vi "configureAcquisition.vi"(6 "imagePaths":path[](array[path]), 7 "saveImages?":bool, 8 "error in (no error)":errorcluster, 9 "number of Images":i32, 10 "CameraSettings":refnum<class "CamaraSettings.lvclass">, 11 "Pixelfly in":refnum<class "Pixelfly.lvclass">) -> (0 "error out":errorcluster, 3 "Pixelfly out":refnum<class "Pixelfly.lvclass">)   [LabVIEW 2009, in "Hardware.lvlib" / "Channels.lvlib" / "Pixelfly.lvclass"]
uses:
  Pixelfly.lvclass
  Tools/CameraSettings/CamaraSettings.lvclass
  Tools/CameraSettings/PixelFlySettings/PixelflySettings.lvclass
  Pixelfly.lvclass/Pixelfly.ctl
  Camera.lvclass
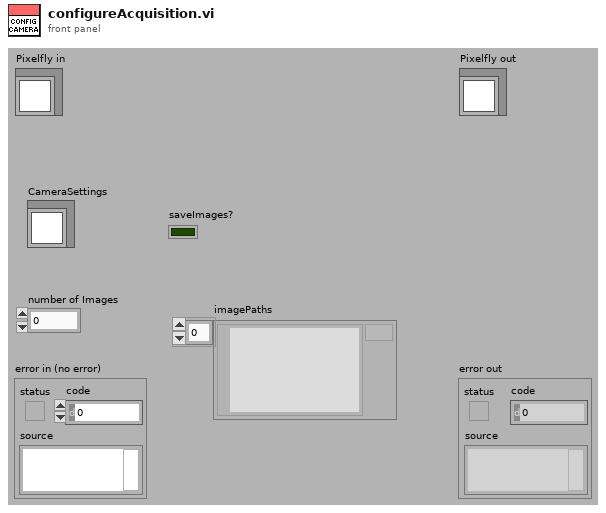
[diagram p1: front panel]
types:
  T1 = cluster{"ccdxsize":i32, "ccdy":i32, "pictx":i32, "picty":i32, "bitspixel":i32}
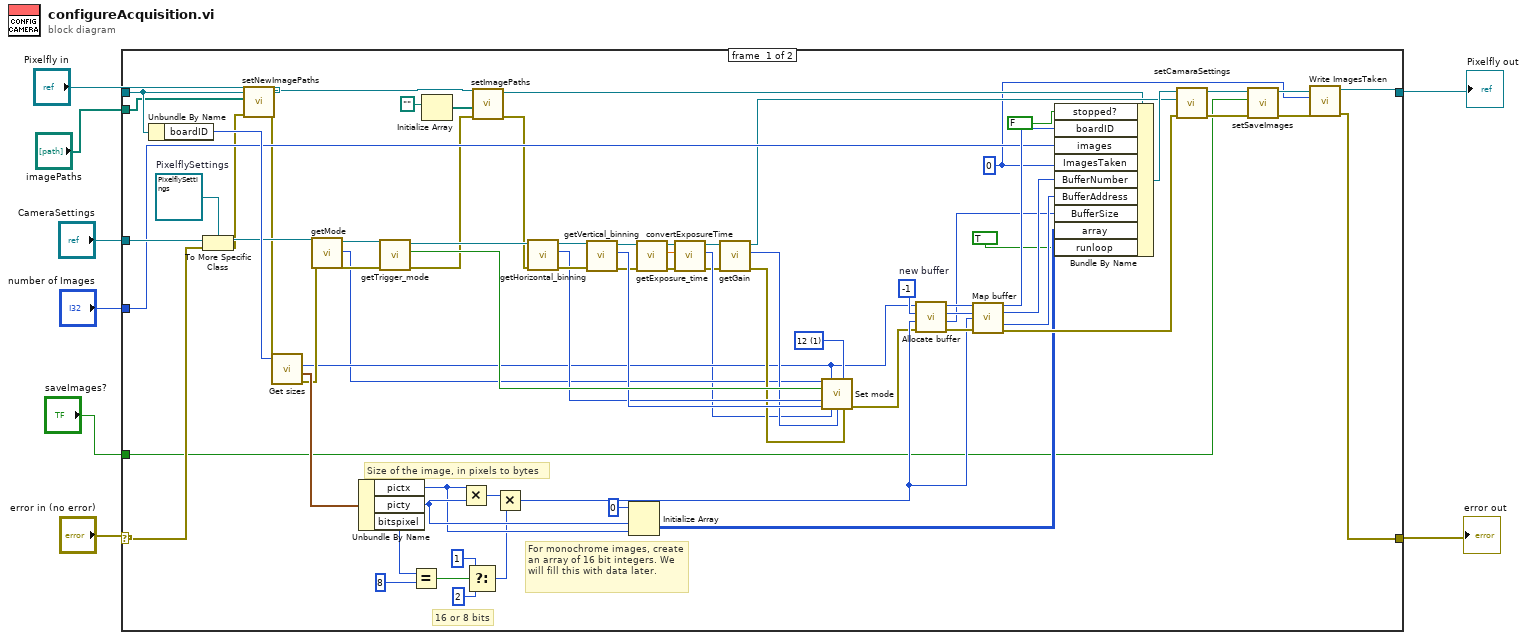
[diagram p0: block diagram]
diagram:
  n1 = case shown="No Error" "error in (no error)" {
    selector: "error in (no error)" -> [w79 w82]
    tunnel: "Pixelfly in" -> [w34 w83]
    tunnel: [w13 w83] -> w4
    tunnel: [w11 w82] -> w3
    tunnel: "CameraSettings" -> [w81 _]
    tunnel: "number of Images" -> [w42 _]
    tunnel: "imagePaths" -> [w31 _]
    tunnel: "saveImages?" -> [w22 _]
    frame #0 {
      w10 = 0
      w60 = 1 items=["8", "12"] ("bits/pixel")
      w63 = -1  # new buffer
      w80 = refnum<class "PixelflySettings.lvclass"> refnum  # PixelflySettings
      # "16 or 8 bits"
      # "For monochrome images, create an array of 16 bit integers. We will fill this with data later."
      # "Size of the image, in pixels to bytes"
      n2 = Unbundle By Name(w34) -> ("boardID"=w61:i32)
      n3 = To More Specific Class(target class=w80, reference=w81, error in=w79) -> (specific class reference=w59:refnum<class "PixelflySettings.lvclass">, error out=w33:errorcluster)
      n4 = call "setNewImagePaths.vi"("error in (no error)"=w33, "NewImagePaths"=w31, "Camera in"=w34) -> ("error out"=w32:errorcluster, "Camera out"=w30:refnum<class "Pixelfly.lvclass">)  [unwired: 7 in]
      n5 = call <instrlib>:"Get sizes.vi"("Handle in"=w61, "error in (no error)"=w32) -> ("Handle out"=w45:i32, "Picture parameters"=w73:T1, "error out"=w58:errorcluster)  [unwired: 1 in, 1 out]
      n6 = call "getMode.vi"("error in (no error)"=w58, "PixelflySettings in"=w59) -> ("error out"=w56:errorcluster, "mode"=w43:u16, "PixelflySettings out"=w57:refnum<class "PixelflySettings.lvclass">)  [unwired: 7 in]
      n7 = Unbundle By Name(w73) -> ("pictx"=w70:i32, "picty"=w71:i32, "bitspixel"=w72:i32)
      n8 = call "getTrigger_mode.vi"("error in (no error)"=w56, "PixelflySettings in"=w57) -> ("error out"=w27:errorcluster, "trigger_mode"=w55:bool, "PixelflySettings out"=w54:refnum<class "PixelflySettings.lvclass">)  [unwired: 7 in]
      n9 = Equal?(x=w72, y=8) -> (x = y?=w69:bool)
      n10 = Initialize Array(path "") -> (w28:path[])  [unwired: 1 in]
      n11 = Multiply(x=w70, y=w71) -> (x*y=w75:i32)
      n12 = Select(t=1, s=w69, f=2) -> (s? t:f=w66:i32)
      n13 = call "setImagePaths.vi"("error in (no error)"=w27, "ImagePaths"=w28, "Camera in"=w30) -> ("error out"=w26:errorcluster, "Camera out"=w25:refnum<class "Pixelfly.lvclass">)  [unwired: 7 in]
      n14 = Multiply(x=w75, y=w66) -> (x*y=w65:i32)
      n15 = call "getHorizontal_binning.vi"("error in (no error)"=w26, "PixelflySettings in"=w54) -> ("error out"=w52:errorcluster, "horizontal_binning"=w50:enum16{"1", "2"}, "PixelflySettings out"=w53:refnum<class "PixelflySettings.lvclass">)  [unwired: 7 in]
      n16 = call "getVertical_binning.vi"("error in (no error)"=w52, "PixelflySettings in"=w53) -> ("error out"=w48:errorcluster, "vertical_binning"=w51:enum16{"1", "2"}, "PixelflySettings out"=w49:refnum<class "PixelflySettings.lvclass">)  [unwired: 7 in]
      n17 = Initialize Array(u16 0 ("16 bit integers"), w71, w70) -> (w35:u16[][])
      n18 = call "getExposure_time.vi"("error in (no error)"=w48, "PixelflySettings in"=w49) -> ("error out"=w17:errorcluster, "exposure_time"=w20:dbl, "PixelflySettings out"=w21:refnum<class "PixelflySettings.lvclass">)  [unwired: 7 in]
      n19 = call "convertExposureTime.vi"("error in (no error)"=w17, "time s"=w20, "PixelflySettings in"=w21) -> ("error out"=w18:errorcluster, "exposureTime"=w19:i32, "PixelflySettings out"=w16:refnum<class "PixelflySettings.lvclass">)  [unwired: 6 in]
      n20 = call "getGain.vi"("error in (no error)"=w18, "PixelflySettings in"=w16) -> ("error out"=w46:errorcluster, "gain"=w47:enum16{"Low", "High"}, "PixelflySettings out"=w37:refnum<class "PixelflySettings.lvclass">)  [unwired: 7 in]
      n21 = call <instrlib>:"Set mode.vi"("Exposure mode"=w43, "Handle in"=w45, "bits/pixel"=w60, "trigger"=w55, "H bin"=w50, "V bin"=w51, "exp time"=w19, "gain"=w47, "error in (no error)"=w46) -> ("error out"=w64:errorcluster)  [unwired: 6 in]
      n22 = call <instrlib>:"Allocate buffer.vi"("error in (no error)"=w64, "Size request"=w65, "Buffer request"=w63, "Handle in"=w45) -> ("error out"=w77:errorcluster, "Size"=w39:i32, "Buffer number"=w62:i32, "Handle out"=w78:i32)
      n23 = call <instrlib>:"Map buffer.vi"("Handle in"=w78, "Buffer in"=w62, "size"=w65, "error in (no error)"=w77) -> ("Handle out"=w44:i32, "Buffer number"=w41:i32, "Buffer address"=w40:i32, "error out"=w36:errorcluster)  [unwired: 8 in]
      n24 = Bundle By Name(cluster=w25, "stopped?"=FALSE, "boardID"=w44, "images"=w42, "ImagesTaken"=w10, "BufferNumber"=w41, "BufferAddress"=w40, "BufferSize"=w39, "array"=w35, "runloop"=TRUE) -> (w38:refnum<class "Pixelfly.lvclass">)
      n25 = call "setCamaraSettings.vi"("error in (no error)"=w36, "CamaraSettings"=w37, "Camera in"=w38) -> ("error out"=w23:errorcluster, "Camera out"=w24:refnum<class "Pixelfly.lvclass">)  [unwired: 7 in]
      n26 = call "setSaveImages.vi"("error in (no error)"=w23, "saveImages?"=w22, "Camera in"=w24) -> ("error out"=w12:errorcluster, "Camera out"=w14:refnum<class "Pixelfly.lvclass">)  [unwired: 7 in]
      n27 = call "Write ImagesTaken.vi"("error in (no error)"=w12, "ImagesTaken"=w10, "Camera in"=w14) -> ("error out"=w11:errorcluster, "Camera out"=w13:refnum<class "Pixelfly.lvclass">)  [unwired: 7 in]
    }
    frame #1 {
    }
  }
  "error out" <- w3
  "Pixelfly out" <- w4
